vi "U Boat main 2.vi"() -> ()   [LabVIEW 2013]
uses:
  <vilib>/Utility/inputDevices.llb/closeJoystick.vi
  <vilib>/Utility/inputDevices.llb/joystickAcquire.vi
panel:
  out "J":u16
  out "R":u16
  out "M":u16
  out "Battery Volts":dbl
  out "Wind Direction":dbl
  out "Wind Speed":dbl
  out "Tilt":dbl
  out "Running?":bool
  in  "Jib Offset":i16(slide) min=-100 max=100 step=1 scale=-100.0..100.0
  in  "Main Offset":i16(slide) min=-100 max=100 step=1 scale=-100.0..100.0
  in  "Manual?":bool=TRUE
  out "Manual Out":i32[](array[numeric])
  in  "VISA resource name":refnum<visa-resource-name>="COM3"
  out "XBee ?":bool
  in  "String":string="$CR1500M1500J1500\n"
  out "bytes written":u32
  out "return count":u32
  out "String Received":string
  in  "Rudder\nOffset":i16(slide) min=-100 max=100 step=1 scale=-100.0..100.0
  out "Jib Sheet":u16=1500
  out "Main sheet":u16=1500
  out "Rudder":u16=1500
  out "error out":errorcluster
  in  "stop":bool
  # "Servo Offsets"
  # "Values without offset"
  # "Raw data from controller"
  # "Initial values"
  # "Values sent"
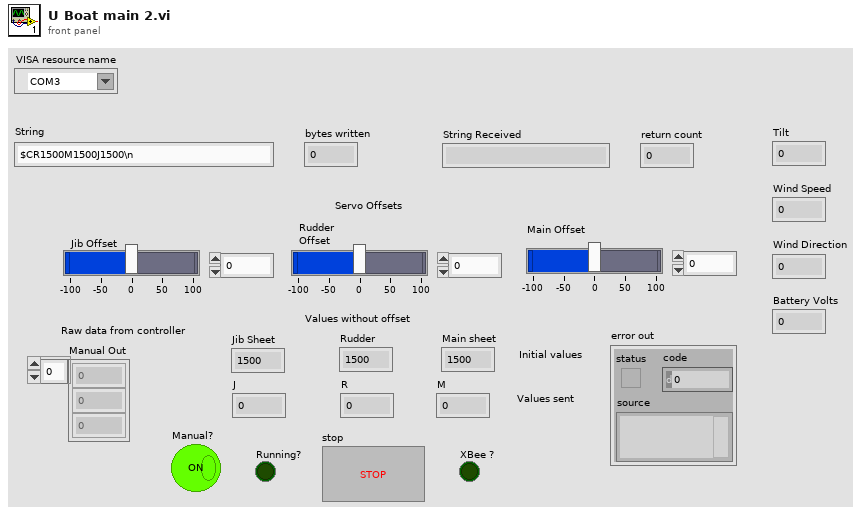
[diagram p1: front panel]
types:
  T1 = cluster{"X axis":i32, "Y axis":i32, "Z axis":i32, "X axis rotation":i32, "Y axis rotation":i32, "Z axis rotation":i32, "U axis":i32, "V axis":i32}
  T2 = cluster{"button 1":bool, "button 2":bool, "button 3":bool, "button 4":bool, "button 5":bool, "button 6":bool, "button 7":bool, "button 8":bool, "button 9":bool, "button 10":bool, "button 11":bool, "button 12":bool, "button 13":bool, "button 14":bool, "button 15":bool, "button 16":bool, "button 17":bool, "button 18":bool, "button 19":bool, "button 20":bool, "button 21":bool, "button 22":bool, "button 23":bool, "button 24":bool, "button 25":bool, "button 26":bool, "button 27":bool, "button 28":bool, "button 29":bool, "button 30":bool, "button 31":bool, "button 32":bool}
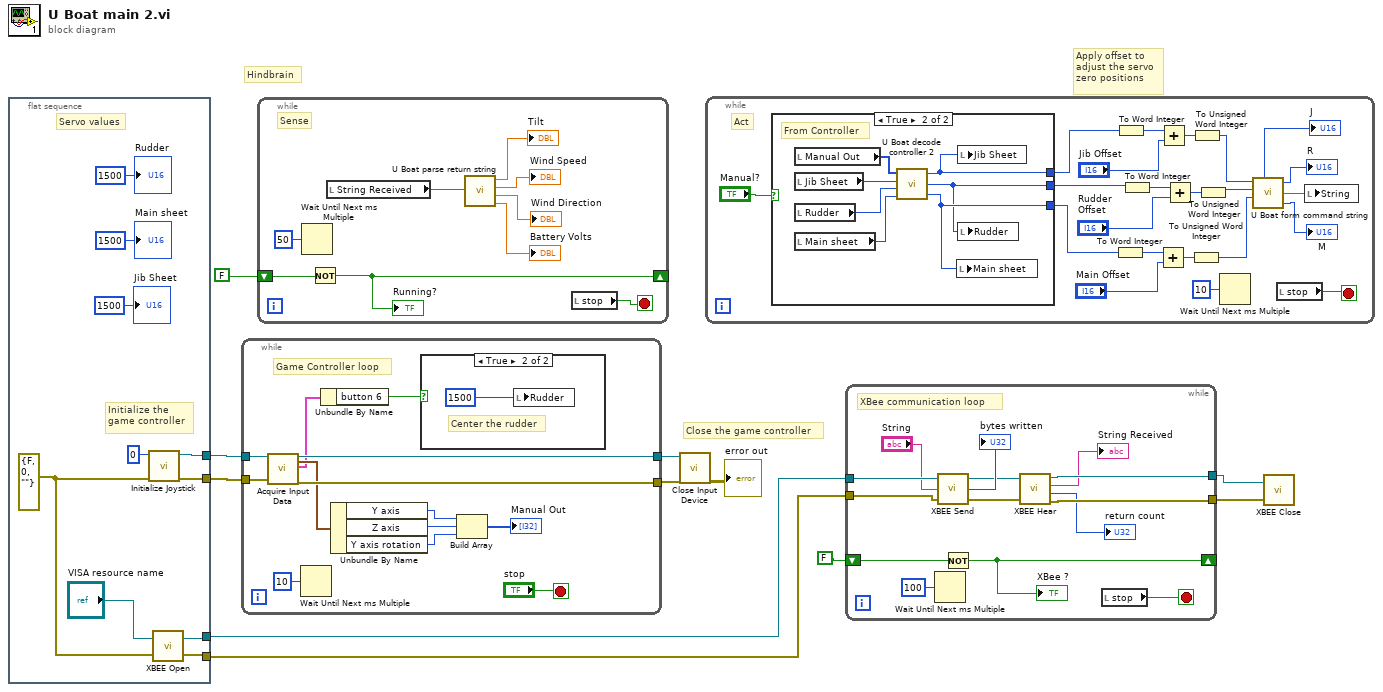
[diagram p0: block diagram]
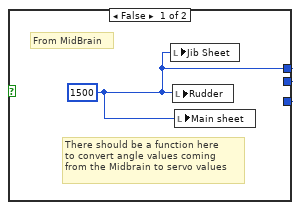
[diagram p2: hidden frame]
diagram:
  # "Apply offset to \nadjust the servo \nzero positions"
  # "Hindbrain"
  # "Close the game controller"
  n1 = flat-sequence {
    tunnel: [w20] -> w11
    tunnel: [w19] -> w9
    tunnel: [w17] -> w4
    tunnel: [w16] -> w3
    frame #0 {
      w12 = errorcluster {"status"=FALSE, "code"=0, "source"=""} ("error in (no error)")
      # "Servo values"
      # "Initialize the\ngame controller"
      n2 = call <vilib>:"Initialize Joystick.vi"("error in (no error)"=w12, "device index"=0) -> ("error out"=w19:errorcluster, "device ID"=w20:refnum<k1>)  [unwired: 8 in]
      n3 = call "XBEE Open.vi"("error in"=w12, "VISA resource name"="VISA resource name") -> ("error out"=w16:errorcluster, "VISA resource name out"=w17:refnum<visa-resource-name>)
      "Rudder" <- u16 1500 ("MRudder")
      "Main sheet" <- u16 1500 ("MRudder")
      "Jib Sheet" <- u16 1500 ("MRudder")
    }
  }
  n4 = while {
    tunnel: w11 -> [w34]
    tunnel: [w33] -> w10
    tunnel: w9 -> [w32]
    tunnel: [w31] -> w8
    stop <- "stop" stop-if-true
    # "Game Controller loop"
    n5 = call-poly <vilib>:"Acquire Input Data.vi"("device ID"=w34, "error in (no error)"=w32) -> ("device ID"=w33:refnum<k1>, "axis info"=w28:T1, "button info"=w23:T2, "error out"=w31:errorcluster)  [unwired: 13 in, 1 out]
    n6 = Wait Until Next ms Multiple(millisecond multiple=u32 10) -> ()  [unwired: 1 out]
    n7 = Unbundle By Name(w23) -> ("button 6"=w22:bool)
    n8 = Unbundle By Name(w28) -> ("Y axis"=w27:i32, "Z axis"=w26:i32, "Y axis rotation"=w25:i32)
    n9 = case shown="True" w22 {
      frame False {
        # "Do nothing"
      }
      frame True {
        # "Center the rudder"
        n10 = local write "Rudder"(u16 1500) -> ()
      }
    }
    n11 = Build Array(w27, w26, w25) -> (→"Manual Out":i32[])
  }
  n12 = while {
    shift-right: [w41] -> _
    shift-left: FALSE -> [w42]
    stop <- w44 stop-if-true
    # "Sense"
    n13 = Wait Until Next ms Multiple(millisecond multiple=u32 50) -> ()  [unwired: 1 out]
    n14 = Not(x=w42) -> (.not. x?=w41:bool)
    "Running?" <- w41
    n15 = local read "String Received"() -> (w40:string)
    n16 = call "U Boat parse return string.vi"("Return String"=w40) -> ("Tilt"=→"Tilt":dbl, "Wind Speed"=→"Wind Speed":dbl, "Wind Direction"=→"Wind Direction":dbl, "Battery Volts"=→"Battery Volts":dbl)
    n17 = local read "stop"() -> (w44:bool)
  }
  n18 = call-poly <vilib>:"Close Input Device.vi"("error in (no error)"=w8, "device ID"=w10) -> ("error out"=→"error out":errorcluster)  [unwired: 8 in]
  n19 = while {
    stop <- w66 stop-if-true
    # "Act"
    n20 = case shown="True" "Manual?" {
      tunnel: [w67 w71] -> w58
      tunnel: [w67 w69] -> w61
      tunnel: [w67 w70] -> w52
      frame False {
        w67 = u16 1500 ("Jib Sheet")
        # "There should be a function here\nto convert angle values coming\nfrom the Midbrain to servo values"
        # "From MidBrain"
        n21 = local write "Jib Sheet"(w67) -> ()
        n22 = local write "Rudder"(w67) -> ()
        n23 = local write "Main sheet"(w67) -> ()
      }
      frame True {
        # "From Controller"
        n24 = local read "Manual Out"() -> (w72:i32[])
        n25 = local read "Jib Sheet"() -> (w73:u16)
        n26 = local read "Rudder"() -> (w68:u16)
        n27 = local read "Main sheet"() -> (w74:u16)
        n28 = call "U Boat decode controller 2.vi"("Main sheet In"=w74, "Rudder In"=w68, "Jib Sheet In"=w73, "Manual In"=w72) -> ("Main sheet Out"=w70:u16, "Rudder Out"=w69:u16, "Jib Steet Out"=w71:u16)
        n29 = local write "Main sheet"(w70) -> ()
        n30 = local write "Jib Sheet"(w71) -> ()
        n31 = local write "Rudder"(w69) -> ()
      }
    }
    n32 = To Word Integer(number=w52) -> (16bit integer=w53:i16)
    n33 = To Word Integer(number=w58) -> (16bit integer=w59:i16)
    n34 = To Word Integer(number=w61) -> (16bit integer=w63:i16)
    n35 = Add(x=w53, y="Main Offset") -> (x+y=w54:i16)
    n36 = Add(x=w59, y="Jib Offset") -> (x+y=w60:i16)
    n37 = Add(x=w63, y="Rudder\nOffset") -> (x+y=w62:i16)
    n38 = To Unsigned Word Integer(number=w54) -> (unsigned 16bit integer=w49:u16)
    n39 = To Unsigned Word Integer(number=w60) -> (unsigned 16bit integer=w51:u16)
    n40 = To Unsigned Word Integer(number=w62) -> (unsigned 16bit integer=w50:u16)
    n41 = Wait Until Next ms Multiple(millisecond multiple=u32 10) -> ()  [unwired: 1 out]
    n42 = call "U Boat form command string.vi"("Jib Sheet"=w51, "Rudder"=w50, "Main sheet"=w49) -> ("Jib"=→"J":u16, "Rudder"=→"R":u16, "String"=w48:string, "Main"=→"M":u16)  [unwired: 1 in]
    n43 = local read "stop"() -> (w66:bool)
    n44 = local write "String"(w48) -> ()
  }
  n45 = while {
    tunnel: w4 -> [w88]
    tunnel: w3 -> [w87]
    tunnel: [w82] -> w6
    tunnel: [w81] -> w5
    shift-right: [w85] -> _
    shift-left: FALSE -> [w86]
    stop <- w75 stop-if-true
    # "XBee communication loop"
    n46 = Wait Until Next ms Multiple(millisecond multiple=u32 100) -> ()  [unwired: 1 out]
    n47 = call "XBEE Send.vi"("error in (no error)"=w87, "String"="String", "VISA resource name"=w88) -> ("error out"=w78:errorcluster, "return count"=→"bytes written":u32, "VISA resource name out"=w79:refnum<visa-resource-name>)
    n48 = Not(x=w86) -> (.not. x?=w85:bool)
    "XBee ?" <- w85
    n49 = call "XBEE Hear.vi"("VISA resource name"=w79, "error in (no error)"=w78) -> ("VISA resource name out"=w82:refnum<visa-resource-name>, "String Received"=→"String Received":string, "return count"=→"return count":u32, "error out"=w81:errorcluster)
    n50 = local read "stop"() -> (w75:bool)
  }
  n51 = call "XBEE Close.vi"("error in (no error)"=w5, "VISA resource name"=w6) -> ()
